vi "AH_FileCheck.vi"(8 "error in":errorcluster, 9 "Config_Cluster":T1={"General"={"Config.ini"=path "", "Default Logging Path"=path ""}, "Hardware"={"AHC VISA COM"="", "Measure Rate (1/s)"=0, "Global T VAR"="", "Global B VAR"="", "Average"=4, "Bias"=0, "Cable"={"Length"=0.0, "Resistance"=0.0, "Inductance"=0.0, "Capacitance"=0.0}, "Tracking"=0, "Voltage"=0.0}, "Operation"={"Operation Mode"=enum."Idle-Off", "Status"="", "NewLog?"=FALSE, "OvenWarn"=FALSE}}, 10 "Exists":bool, 11 "Path IN":path) -> (0 "error Out":errorcluster, 1 "Config_Cluster Out":T1={"General"={"Config.ini"=path "", "Default Logging Path"=path ""}, "Hardware"={"AHC VISA COM"="", "Measure Rate (1/s)"=0, "Global T VAR"="", "Global B VAR"="", "Average"=4, "Bias"=0, "Cable"={"Length"=0.0, "Resistance"=0.0, "Inductance"=0.0, "Capacitance"=0.0}, "Tracking"=0, "Voltage"=0.0}, "Operation"={"Operation Mode"=enum."Idle-Off", "Status"="", "NewLog?"=FALSE, "OvenWarn"=FALSE}}, 2 "Continue":bool, 3 "refnum":refnum<file>)   [LabVIEW 2021]
uses:
  Config_Cluster.ctl
  Mode_Enum.ctl
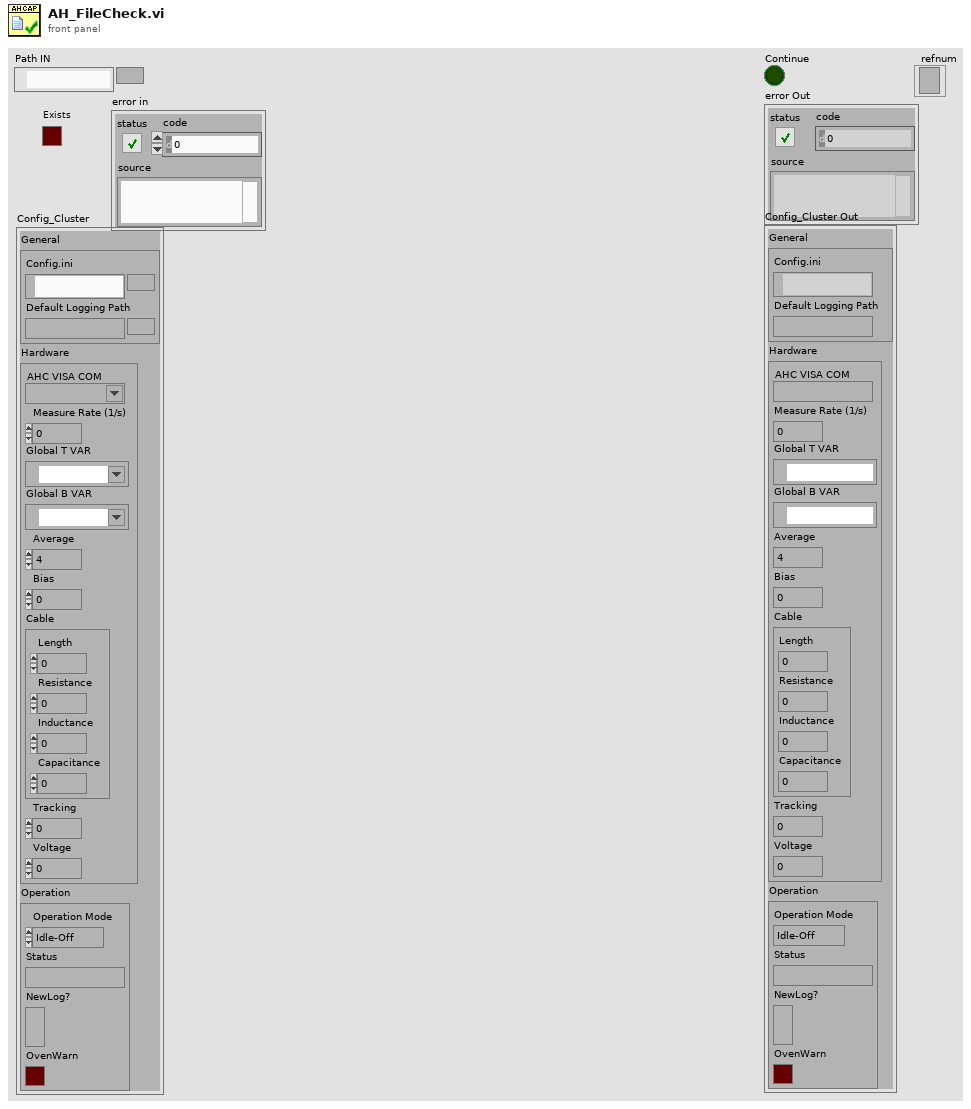
[diagram p1: front panel]
types:
  T1 = typedef "Config_Cluster.ctl" = cluster{"General":cluster{"Config.ini":path, "Default Logging Path":path}, "Hardware":cluster{"AHC VISA COM":refnum<visa-resource-name>, "Measure Rate (1/s)":i32, "Global T VAR":refnum<k21>, "Global B VAR":refnum<k21>, "Average":u8, "Bias":u8, "Cable":cluster{"Length":dbl, "Resistance":dbl, "Inductance":dbl, "Capacitance":dbl}, "Tracking":u8, "Voltage":dbl}, "Operation":cluster{"Operation Mode":T2, "Status":string, "NewLog?":bool, "OvenWarn":bool}}
  T2 = typedef "Mode_Enum.ctl" = enum16{"OvenNRDY", "Logging", "Idle-Off", "Idle"}
  T3 = enum16{"open", "replace", "create", "open or create", "replace or create", "replace or create with confirmation"}
  T4 = enum16{"Left Button", "Center Button", "Right Button", "Window Close"}
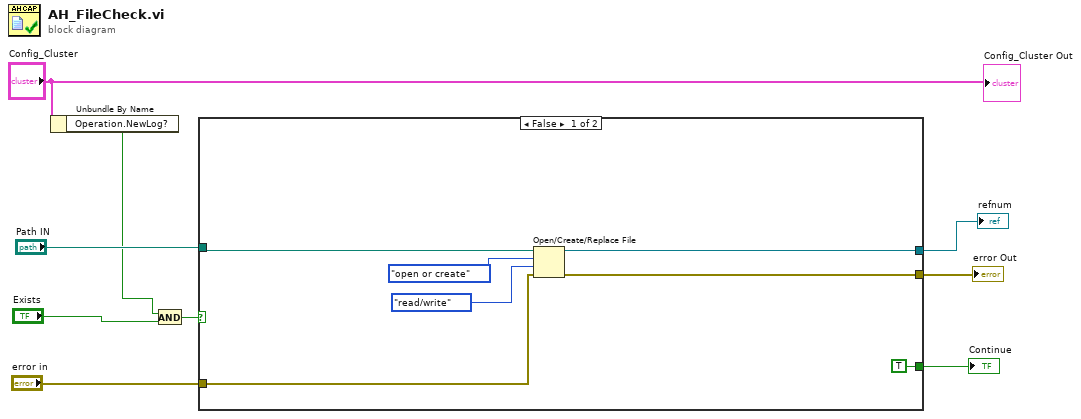
[diagram p0: block diagram]
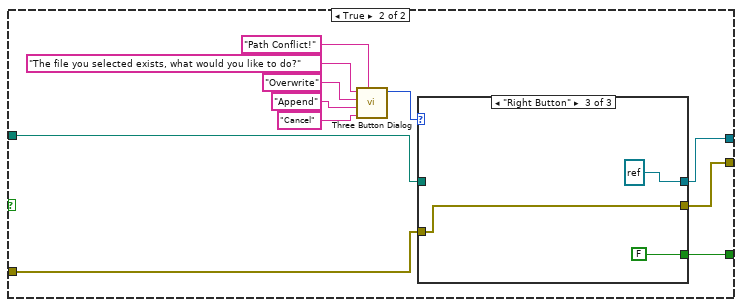
[diagram p2: hidden frame]
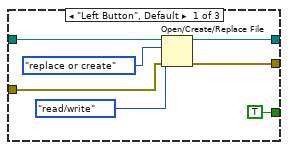
[diagram p3: hidden frame]
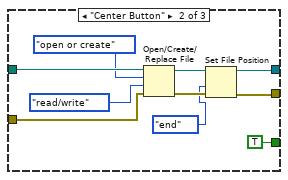
[diagram p4: hidden frame]
diagram:
  n1 = Unbundle By Name("Config_Cluster") -> ("Operation.NewLog?"=w1:bool)
  n2 = And(x=w1, y="Exists") -> (x .and. y?=w3:bool)
  n3 = case shown="False" w3 {
    tunnel: "Path IN" -> [w16 w21]
    tunnel: "error in" -> [w13 w20]
    tunnel: [w12 w19] -> w5
    tunnel: [w11 w18] -> w6
    tunnel: [TRUE w17] -> w7
    frame False {
      n4 = Open/Create/Replace File(file path (use dialog)=w16, error in=w13, operation (0:open)=T3."open or create", access (0:read/write)=enum16{"read/write", "read-only", "write-only"}."read/write") -> (refnum out=w12:refnum<file>, error out=w11:errorcluster)  [unwired: 2 in, 1 out]
    }
    frame True {
      n5 = call <vilib>:"Three Button Dialog.vi"("Window Title (\"\")"="Path Conflict!" ("Window Title (\"\")"), "Right Button Text (\"Cancel\")"="Cancel" ("Right Button Text (\"Cancel\")"), "Center Button Text (\"No\")"="Append" ("Center Button Text (\"No\")"), "Left Button Text (\"Yes\")"="Overwrite" ("Left Button Text (\"Yes\")"), "message"="The file you selected exists, what would you like to do?") -> ("Which Button?"=w22:T4)  [unwired: 6 in]
      n6 = case shown="\"Right Button\"" w22 {
        tunnel: w21 -> [w34 w44 _]
        tunnel: w20 -> [w33 w43 w46]
        tunnel: [w30 w41 refnum<file> refnum ("refnum")] -> w19
        tunnel: [w29 w40 w46] -> w18
        tunnel: [TRUE TRUE FALSE] -> w17
        frame "Left Button", Default {
          n7 = Open/Create/Replace File(file path (use dialog)=w34, error in=w33, operation (0:open)=T3."replace or create", access (0:read/write)=enum16{"read/write", "read-only", "write-only"}."read/write") -> (refnum out=w30:refnum<file>, error out=w29:errorcluster)  [unwired: 2 in, 1 out]
        }
        frame "Center Button" {
          n8 = Open/Create/Replace File(file path (use dialog)=w44, error in=w43, operation (0:open)=T3."open or create", access (0:read/write)=enum16{"read/write", "read-only", "write-only"}."read/write") -> (refnum out=w42:refnum<file>, error out=w39:errorcluster)  [unwired: 2 in, 1 out]
          n9 = Set File Position(refnum=w42, from (0:start)=enum16{"start", "end", "current"}."end", error in=w39) -> (refnum out=w41:refnum<file>, error out=w40:errorcluster)  [unwired: 1 in]
        }
        frame "Right Button" {
        }
      }
    }
  }
  "Continue" <- w7
  "error Out" <- w6
  "refnum" <- w5
  "Config_Cluster Out" <- "Config_Cluster"
